vi "Write Status Display.vi"(8 "error in (no error)":errorcluster, 10 "Status Display":refnum<vi>, 11 "Function UI in":refnum<class "Controller UI.lvclass">) -> (0 "error out":errorcluster, 3 "Function UI out":refnum<class "Controller UI.lvclass">)   [LabVIEW 2016, in "Controller UI.lvlib" / "Controller UI.lvclass"]
uses:
  <userlib>/Common Components/Controller UI/Controller UI.lvclass
  <userlib>/Common Components/Controller UI/Controller UI.lvclass/Controller UI.ctl
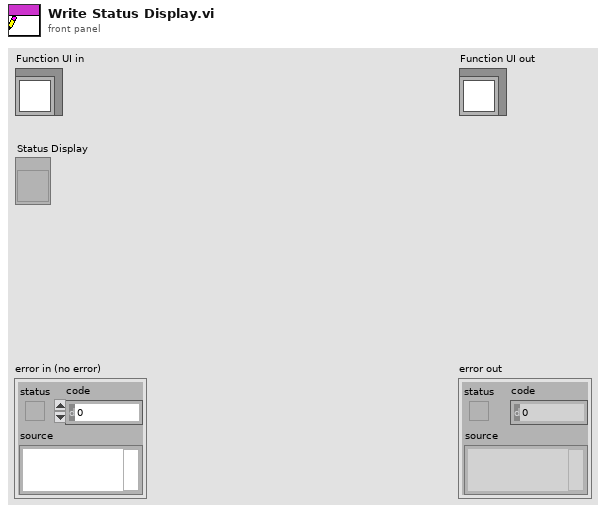
[diagram p1: front panel]
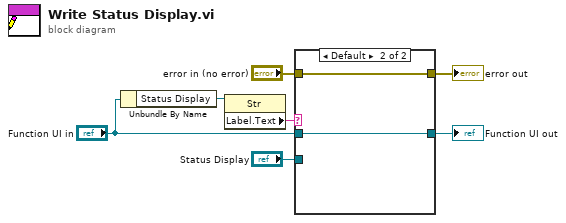
[diagram p0: block diagram]
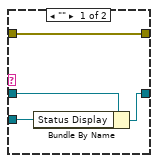
[diagram p2: hidden frame]
diagram:
  n1 = Unbundle By Name("Function UI in") -> ("Status Display"=w2:refnum<vi>)
  n2 = property class="Str"(reference=w2) -> ("Label.Text"=w1:string)  [unwired: 1 in, 2 out]
  n3 = case shown="Default" w1 {
    tunnel: [w8 w12] -> w7
    tunnel: [w10 w13] -> w6
    tunnel: "Function UI in" -> [w11 w13]
    tunnel: "Status Display" -> [w9 _]
    tunnel: "error in (no error)" -> [w8 w12]
    frame "" {
      n4 = Bundle By Name(cluster=w11, "Status Display"=w9) -> (w10:refnum<class "Controller UI.lvclass">)
    }
    frame Default {
    }
  }
  "error out" <- w7
  "Function UI out" <- w6
